vi "phase correction.vi"(1 "Deg/Rad":enum16{"Rad", "Deg"}(ring), 2 "Complex FFT":cdb[](array[numeric])) -> (0 "Phase":dbl[](array[numeric]))   [LabVIEW 2009]
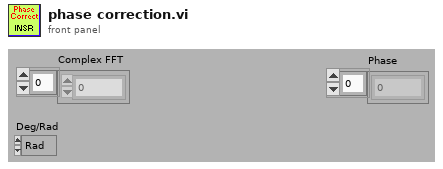
[diagram p1: front panel]
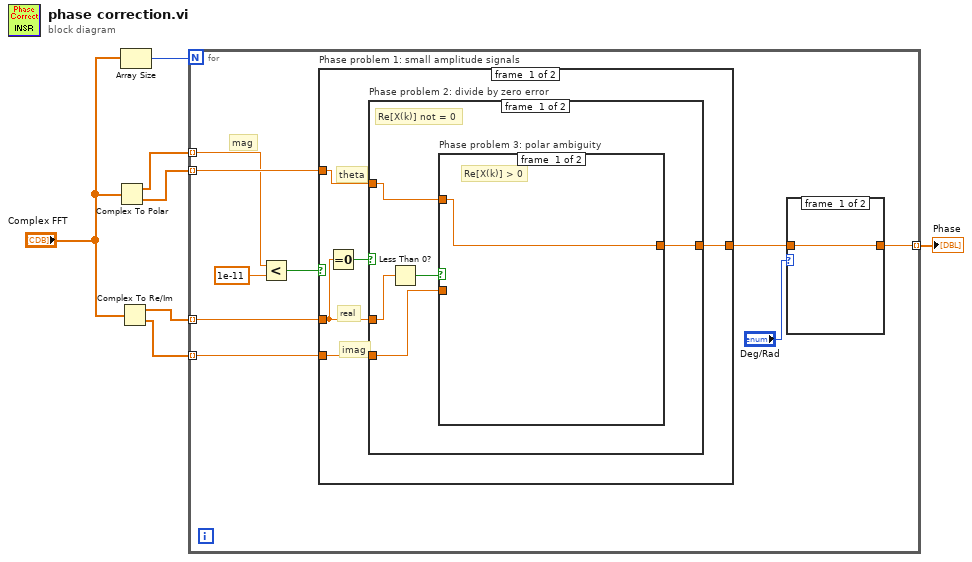
[diagram p0: block diagram]
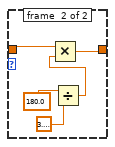
[diagram p2: hidden frame]
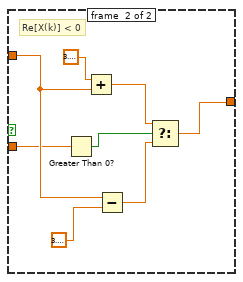
[diagram p3: hidden frame]
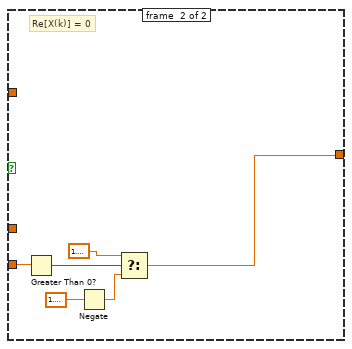
[diagram p4: hidden frame]
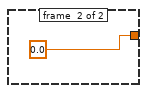
[diagram p5: hidden frame]
diagram:
  n1 = Complex To Polar(r * e^(i*theta)="Complex FFT") -> (r=w7:dbl[], theta=w6:dbl[])
  n2 = Complex To Re/Im(x + iy="Complex FFT") -> (x=w4:dbl[], y=w5:dbl[])
  n3 = Array Size(array="Complex FFT") -> (size(s)=w2:i32)
  n4 = for {
    N: w2 -> [_]
    tunnel: w7 -> [w13] mode=indexing
    tunnel: w6 -> [w16] mode=indexing
    tunnel: w5 -> [w15] mode=indexing
    tunnel: w4 -> [w14] mode=indexing
    tunnel: [w9] -> w1 mode=indexing
    # "mag"
    n5 = Less?(x=w13, y=1e-11) -> (x < y?=w11:bool)
    n6 = case "Phase problem 1: small amplitude signals" shown="False" w11 {
      tunnel: w16 -> [w27 _]
      tunnel: w15 -> [w26 _]
      tunnel: w14 -> [w25 _]
      tunnel: [w23 0.0] -> w10
      frame #0 {
        # "imag"
        # "real"
        # "theta"
        n7 = Equal To 0?(x=w25) -> (x = 0?=w24:bool)
        n8 = case "Phase problem 2: divide by zero error" shown="False" w24 {
          tunnel: w27 -> [w30 _]
          tunnel: w25 -> [w32 _]
          tunnel: w26 -> [w28 w47]
          tunnel: [w29 w42] -> w23
          frame #0 {
            # "Re[X(k)] not = 0"
            n9 = Less Than 0?(x=w32) -> (x < 0?=w31:bool)
            n10 = case "Phase problem 3: polar ambiguity" shown="True" w31 {
              tunnel: w30 -> [w33 w38]
              tunnel: [w33 w34] -> w29
              tunnel: w28 -> [_ w35]
              frame #0 {
                # "Re[X(k)] > 0"
              }
              frame #1 {
                # "Re[X(k)] < 0"
                n11 = Greater Than 0?(x=w35) -> (x > 0?=w36:bool)
                n12 = Add(x=3.141592653589793, y=w38) -> (x+y=w37:dbl)
                n13 = Subtract(x=w38, y=3.141592653589793) -> (x-y=w39:dbl)
                n14 = Select(t=w37, s=w36, f=w39) -> (s? t:f=w34:dbl)
              }
            }
          }
          frame #1 {
            # "Re[X(k)] = 0"
            n15 = Greater Than 0?(x=w47) -> (x > 0?=w46:bool)
            n16 = Negate(x=1.5707963267948966) -> (-x=w43:dbl)
            n17 = Select(t=1.5707963267948966, s=w46, f=w43) -> (s? t:f=w42:dbl)
          }
        }
      }
      frame #1 {
      }
    }
    n18 = case shown="\"Deg\"" "Deg/Rad" {
      tunnel: w10 -> [w17 w20]
      tunnel: [w17 w18] -> w9
      frame #0 {
      }
      frame #1 {
        n19 = Divide(x=180.0 ("y"), y=3.141592653589793) -> (x/y=w19:dbl)
        n20 = Multiply(x=w20, y=w19) -> (x*y=w18:dbl)
      }
    }
  }
  "Phase" <- w1
